vi "Main.vi"() -> ()   [LabVIEW 2013]
uses:
  <vilib>/myRIO/Instrument Drivers/Onboard IO/I2C/typedefs/I2C User Configuration.ctl
  <vilib>/myRIO/Instrument Drivers/Onboard IO/I2C/typedefs/I2C Transfer Rate.ctl
  <vilib>/Platform/TimedLoop/XDataNode/timing_clust.ctl
  <vilib>/Platform/TimedLoop/XDataNode/nitl_modes.ctl
  <vilib>/Platform/TimedLoop/XDataNode/wakeup.ctl
  <vilib>/myRIO/Common/Instrument Driver Framework/myRIO v1.0/I2C/vis/myRIO v1.1 Open I2C.vi
  <vilib>/myRIO/Common/Instrument Driver Framework/myRIO v1.0/UART/vis/myRIO v1.0 Close UART.vi
  <vilib>/myRIO/Common/Instrument Driver Framework/Utilities/vis/Validate Channels.vi
  <vilib>/myRIO/Common/Instrument Driver Framework/myRIO v1.0/I2C/vis/myRIO v1.0 Reserve I2C.vi
  <vilib>/myRIO/Common/Instrument Driver Framework/myRIO v1.0/I2C/vis/myRIO v1.0 Build MUX Configuration I2C.vi
  <vilib>/myRIO/Common/Instrument Driver Framework/myRIO v1.0/Resource Manager/vis/myRIO v1.0 Reserve Channel List.vi
  <vilib>/myRIO/Common/Instrument Driver Framework/myRIO v1.0/Resource Manager/vis/myRIO v1.0 Create Configuration List.vi
  <vilib>/myRIO/Common/Instrument Driver Framework/myRIO v1.0/Resource Manager/vis/myRIO v1.0 Reserve Channel.vi
  <vilib>/myRIO/Common/Instrument Driver Framework/myRIO v1.0/Resource Manager/vis/myRIO v1.0 Unreserve Channel.vi
  <vilib>/myRIO/Common/Instrument Driver Framework/myRIO v1.0/Resource Manager/vis/myRIO v1.0 Build Mutex Name.vi
  <vilib>/myRIO/Common/Instrument Driver Framework/myRIO v1.0/myRIO v1.1 Open.vi
  <vilib>/Utility/VariantDataType/GetNumericInfo.vi
  <vilib>/Utility/error.llb/Error Cluster From Error Code.vi
  <vilib>/myRIO/Common/Instrument Driver Framework/Utilities/vis/IO Manager.vi
  <vilib>/myRIO/Common/Instrument Driver Framework/Utilities/vis/Configuration Manager.vi
  <vilib>/myRIO/Common/Instrument Driver Framework/myRIO v1.0/Resource Manager/vis/myRIO v1.0 Configure IO.vi
  <vilib>/myRIO/Common/Instrument Driver Framework/myRIO v1.0/myRIO v1.0 Close.vi
  <vilib>/myRIO/Common/Instrument Driver Framework/myRIO v1.0/I2C/vis/myRIO v1.0 Configure I2C.vi
  <vilib>/myRIO/Common/Instrument Driver Framework/myRIO v1.0/I2C/vis/myRIO v1.0 Write I2C.vi
  <vilib>/myRIO/Common/Instrument Driver Framework/myRIO v1.0/I2C/vis/myRIO v1.0 Read I2C.vi
  <vilib>/myRIO/Common/Instrument Driver Framework/Utilities/vis/FPGA Ref Manager.vi
  <vilib>/myRIO/Common/Instrument Driver Framework/myRIO v1.0/myRIO v1.0 Reset FPGA.vi
  <vilib>/platform/TimedLoop/XDataNode/XDataNode.xnode
  <vilib>/myRIO/Instrument Drivers/Utilities/Utilities.lvlib
  <vilib>/myRIO/Instrument Drivers/Onboard IO/I2C/I2C.lvlib
  <vilib>/Platform/TimedLoop/XDataNode/XDNodeRunTimeDep.lvlib
panel:
  out "Waveform Chart":cluster{i16, i16, i16}(graph)
  out "Z":i16
  out "Y":i16
  out "X":i16
  in  "[ESC]":bool
  # "DATAX0"
  # "DATAX1"
  # "DATAY0"
  # "DATAY1"
  # "DATAZ0"
  # "DATAZ1"
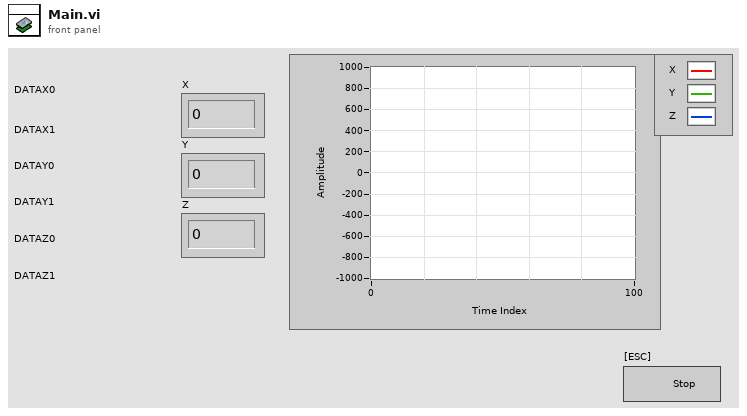
[diagram p1: front panel]
types:
  T1 = typedef "I2C.lvlib/I2C User Configuration.ctl" = cluster{"I2C Transfer Rate":T2}
  T2 = typedef "I2C.lvlib/I2C Transfer Rate.ctl" = enum16{"Standard Mode (100 kbps)", "Fast Mode (400 kbps)"}
  T3 = typedef "I2C.lvlib/I2C Reference.ctl" = cluster{"myRIO Reference":T4, "I2C Channels Enum":T8, "I2C Configuration":T9}
  T4 = typedef "myRIO Generic Hardware Reference.ctl" = cluster{"myRIO Model":T5, "myRIO Hardware Reference":T6}
  T5 = typedef "Hardware Version Enum.ctl" = enum16{"Unknown", "myRIO-1900", "myRIO-1950"}
  T6 = typedef "myRIO v1.0 Reference.ctl" = cluster{"Generic FPGA Reference":T7, "Allow multiple opens":bool}
  T7 = typedef "Generic FPGA Reference.ctl" = refnum<k20>
  T8 = typedef "I2C Channels Enum.ctl" = enum16{"Not Connected", "A/I2C", "B/I2C"}
  T9 = typedef "I2C.lvlib/I2C Configuration.ctl" = cluster{"I2C Transfer Rate":T2}
  T10 = typedef "XDNodeRunTimeDep.lvlib/timing_clust.ctl" = cluster{"Expected End [f-1]":u64, "Actual End [f-1]":u64, "Finished Late? [f-1]":bool, "Expected End [i-1]":u64, "Actual End [i-1]":u64, "Finished Late? [i-1]":bool, "Expected Start [i]":u64, "Actual Start [i]":u64, "Expected Start [f]":u64, "Actual Start [f]":u64, "Source Name":string, "Structure Name":string, "Period":i64, "Deadline":i64, "Offset":i64, "Start":i64, "Priority":i32, "Timeout":i32, "Mode":T11, "Wakeup Reason":T12, "Error":errorcluster, "Source Type":string, "Secondary Source Type":string, "Global End Time":u64, "Global Start Time":u64, "Frame Duration":u64, "Iteration Duration":u64, "Assigned CPU":i32, "I/O Scan Engine Mode":u32}
  T11 = typedef "XDNodeRunTimeDep.lvlib/nitl_modes.ctl" = enum32{"No Change", "Process missed periods, maintain original phase", "Discard missed periods, maintain original phase", "Process missed periods, ignore original phase", "Discard missed periods, ignore original phase"}
  T12 = typedef "XDNodeRunTimeDep.lvlib/wakeup.ctl" = enum32{"Normal", "Aborted", "Asynchronous wakeup", "Timing source error", "Timed loop error", "Timeout"}
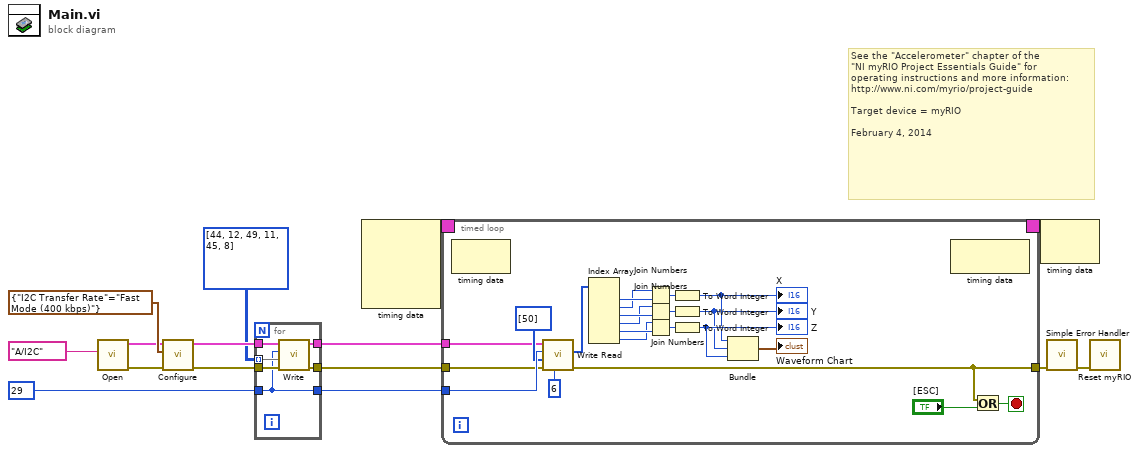
[diagram p0: block diagram]
diagram:
  # "See the \"Accelerometer\" chapter of the\n\"NI myRIO Project Essentials Guide\" for\noperating instructions and more information: \nhttp://www.ni.com/myrio/project-guide\n\nTarget device = myRIO\n\nFebruary 4, 2014"
  n1 = call <vilib>:"Open.vi"("Channel Name"=tag "A/I2C" ("I2C channel")) -> ("error out"=w11:errorcluster, "I2C Ref Out"=w12:T3)  [unwired: 9 in]
  n2 = call <vilib>:"Configure.vi"("error in (no error)"=w11, "I2C User Configuration"=T1 {"I2C Transfer Rate"=enum."Fast Mode (400 kbps)"} ("I2C bus speed"), "I2C Ref In"=w12) -> ("error out"=w6:errorcluster, "I2C Ref Out"=w7:T3)  [unwired: 7 in]
  n3 = for {
    tunnel: [w21] -> w10
    tunnel: [w20] -> w9
    tunnel: [w16] -> w8
    tunnel: u8[][] [[44, 12], [49, 11], [45, 8]] ("Bytes to Write") -> [w19] mode=indexing
    tunnel: w7 -> [w18]
    tunnel: w6 -> [w17]
    tunnel: u8 29 ("PmodACL") -> [w16]
    n4 = call <vilib>:"Write.vi"("error in (no error)"=w17, "Bytes to Write"=w19, "Slave Address (7-bit)"=w16, "I2C Ref In"=w18) -> ("error out"=w21:errorcluster, "I2C Ref Out"=w20:T3)  [unwired: 6 in]
  }
  n5 = node-c288() -> (w4:T10)  [unwired: 4 in]
  n6 = timed-loop {
    tunnel: w8 -> [w41]
    tunnel: w10 -> [w23]
    tunnel: w9 -> [w24]
    timing: w4 -> [_]
    timing-out: [_] -> w3
    tunnel: [w22] -> w1
    stop <- w43 stop-if-true
    n7 = node-c288() -> ()  [unwired: 1 in, 1 out]
    n8 = call <vilib>:"Write Read.vi"("Byte Count"=u32 6, "error in (no error)"=w23, "Bytes to Write"=u8[] [50], "Slave Address (7-bit)"=w41, "I2C Ref In"=w24) -> ("error out"=w22:errorcluster, "Bytes Read"=w25:u8[])  [unwired: 3 in, 1 out]
    n9 = Index Array(array=w25) -> (element #1=w33:u8, element #2=w32:u8, element #3=w31:u8, element #4=w30:u8, element #5=w29:u8, element #6=w28:u8)  [unwired: 6 in]
    n10 = Join Numbers(hi=w32, lo=w33) -> ((hi.lo)=w40:u16)
    n11 = Join Numbers(hi=w30, lo=w31) -> ((hi.lo)=w39:u16)
    n12 = Join Numbers(hi=w28, lo=w29) -> ((hi.lo)=w38:u16)
    n13 = To Word Integer(number=w40) -> (16bit integer=w35:i16)
    "X" <- w35
    n14 = To Word Integer(number=w39) -> (16bit integer=w34:i16)
    "Y" <- w34
    n15 = To Word Integer(number=w38) -> (16bit integer=w37:i16)
    "Z" <- w37
    n16 = Bundle(w35, w34, w37) -> (→"Waveform Chart":cluster{i16, i16, i16})  [unwired: 1 in]
    n17 = node-c288() -> ()  [unwired: 1 in, 1 out]
    n18 = Or(x=w22, y="[ESC]") -> (x .or. y?=w43:bool)
  }
  n19 = node-c288(w3) -> ()  [unwired: 1 out]
  n20 = call <vilib>:"Simple Error Handler.vi"("error in (no error)"=w1) -> ("error out"=w15:errorcluster)  [unwired: 4 in, 4 out]
  n21 = call <vilib>:"Reset myRIO.vi"("error in (no error)"=w15) -> ()  [unwired: 10 in, 1 out]
